vi "TrALEX_RNG.vi"(0 "Analog Amplitude":dbl=1.0 format="%0.2p", 1 "Repetition Frequency":dbl=2.0 format="%.6f") -> ()   [LabVIEW 2011]
uses:
  <vilib>/DAQmx/write.llb/DAQmx Write (Analog Wfm 1Chan NSamp).vi
  <vilib>/DAQmx/create/channels.llb/DAQmx Create Channel (AO-Voltage-Basic).vi
  <vilib>/DAQmx/configure/timing.llb/DAQmx Timing (Sample Clock).vi
  <vilib>/DAQmx/create/channels.llb/DAQmx Create Channel (CO-Pulse Generation-Frequency).vi
  <vilib>/DAQmx/configure/events/hardwareSignals.llb/DAQmx Export Signal (Most Signals).vi
  <vilib>/DAQmx/configure/trigger.llb/DAQmx Start Trigger (Digital Edge).vi
  <vilib>/DAQmx/configure/timing.llb/DAQmx Timing (Implicit).vi
  <vilib>/DAQmx/miscellaneous.llb/DAQmx Fill In Error Info.vi
  <vilib>/measure/NI_MABase.lvlib
panel:
  in  "Three Colour Duty Cycle":dbl=0.3333333333333333 format="%.6f"
  in  "Stop Button":bool
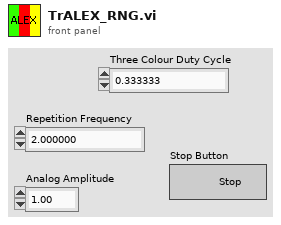
[diagram p1: front panel]
types:
  T1 = enum16{"Sine Wave", "Triangle Wave", "Square Wave", "Sawtooth Wave"}
  T2 = cluster{"Ao0 Sample Clock Rate":dbl, "Ao0 Sample Clock Rate":dbl}
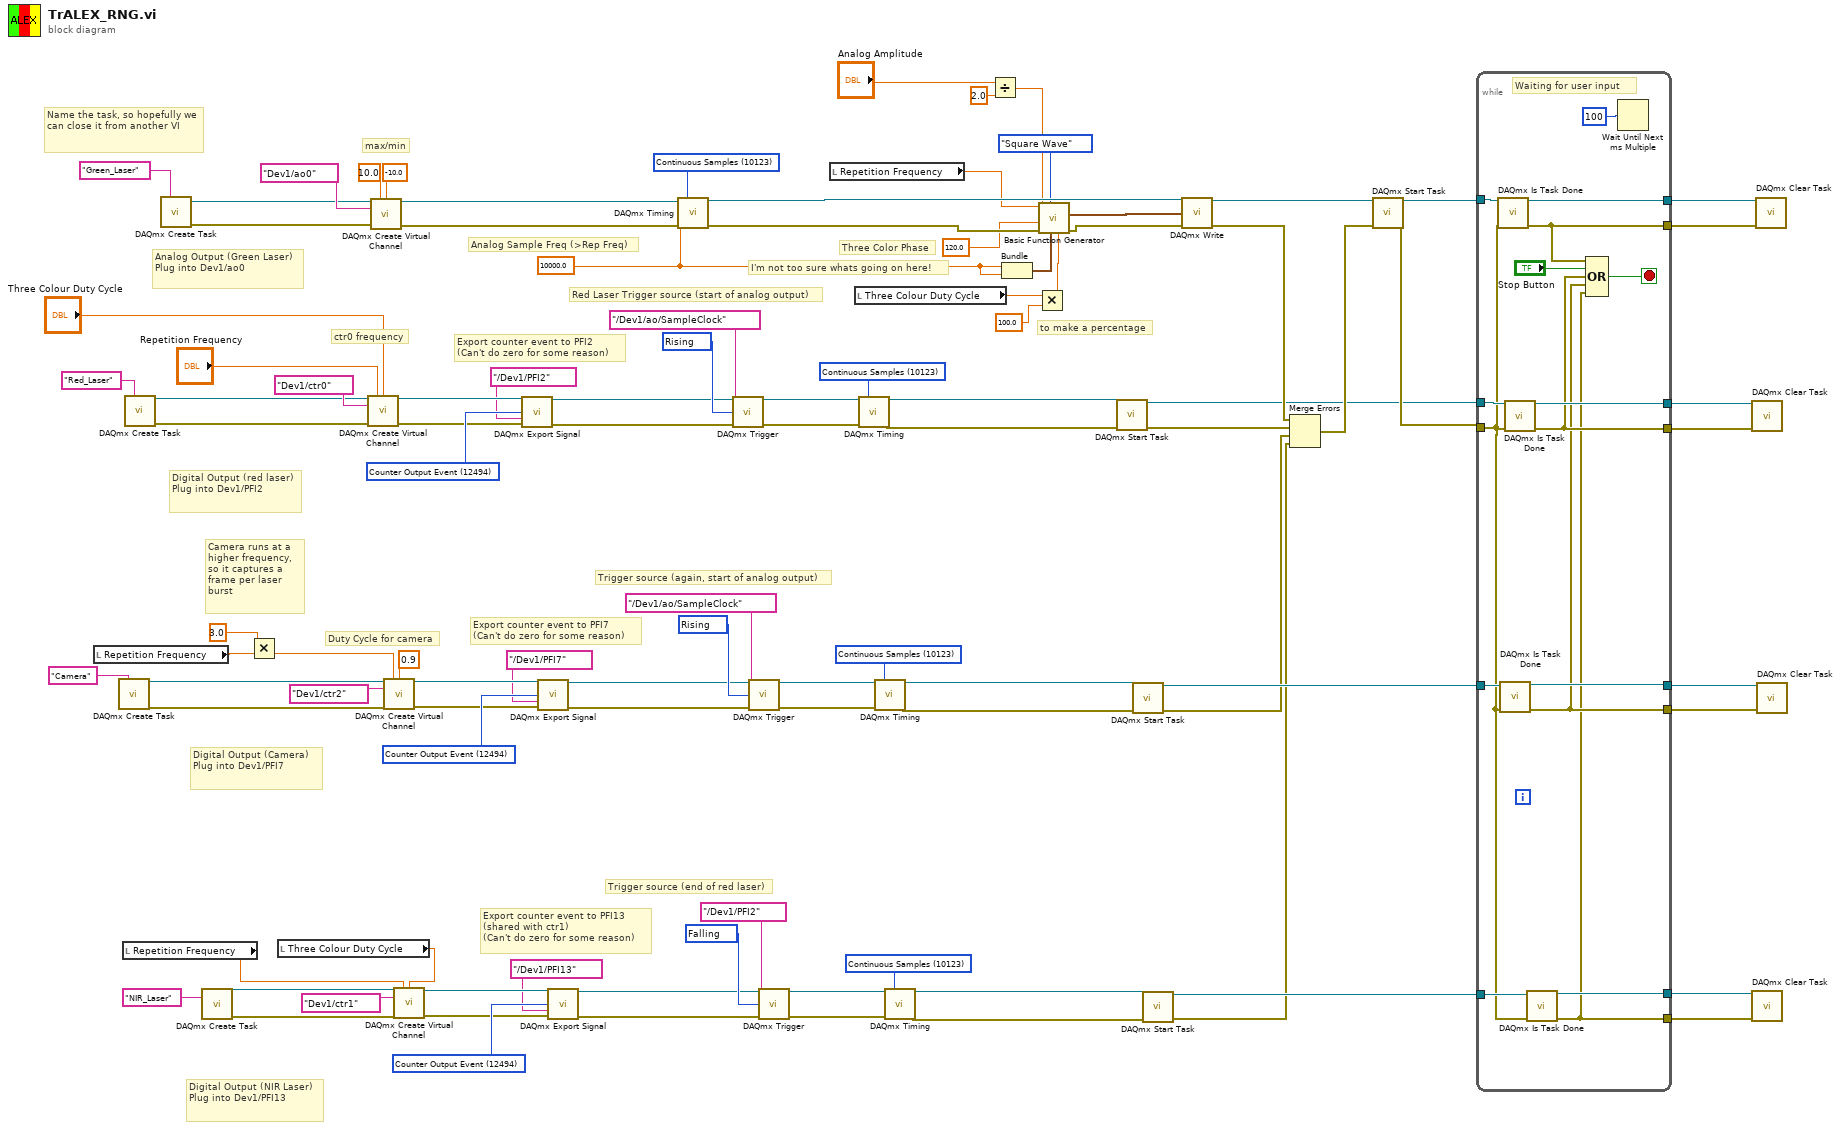
[diagram p0: block diagram]
diagram:
  w30 = 10171 items=["Rising"=10280, "Falling"=10171] ("edge")
  w33 = 10123 items=["Finite Samples"=10178, "Continuous Samples"=10123, "Hardware Timed Single Point"=12522] ("sample mode")
  w35 = 12494 items=["AI Convert Clock"=12484, "10MHz Reference Clock"=12536, "20MHz Timebase Clock"=12486, "Sample Clock"=12487, "Advance Trigger"=12488, "Reference Trigger"=12490, "Start Trigger"=12491, "Advance Complete Event"=12492, "AI Hold Complete Event"=12493, "Counter Output Event"=12494, "Change Detection Event"=12511, "Watchdog Timer Expired Event"=12512] ("signal")
  w54 = 10280 items=["Rising"=10280, "Falling"=10171] ("edge")
  w57 = 10123 items=["Finite Samples"=10178, "Continuous Samples"=10123, "Hardware Timed Single Point"=12522] ("sample mode")
  w59 = 12494 items=["AI Convert Clock"=12484, "10MHz Reference Clock"=12536, "20MHz Timebase Clock"=12486, "Sample Clock"=12487, "Advance Trigger"=12488, "Reference Trigger"=12490, "Start Trigger"=12491, "Advance Complete Event"=12492, "AI Hold Complete Event"=12493, "Counter Output Event"=12494, "Change Detection Event"=12511, "Watchdog Timer Expired Event"=12512] ("signal")
  w68 = 10123 items=["Finite Samples"=10178, "Continuous Samples"=10123, "Hardware Timed Single Point"=12522] ("sample mode")
  w89 = 10280 items=["Rising"=10280, "Falling"=10171] ("edge")
  w94 = 10123 items=["Finite Samples"=10178, "Continuous Samples"=10123, "Hardware Timed Single Point"=12522] ("sample mode")
  w96 = 12494 items=["AI Convert Clock"=12484, "10MHz Reference Clock"=12536, "20MHz Timebase Clock"=12486, "Sample Clock"=12487, "Advance Trigger"=12488, "Reference Trigger"=12490, "Start Trigger"=12491, "Advance Complete Event"=12492, "AI Hold Complete Event"=12493, "Counter Output Event"=12494, "Change Detection Event"=12511, "Watchdog Timer Expired Event"=12512] ("signal")
  w37 = 10000.0 ("Ao0 Sample Clock Rate")
  # "Name the task, so hopefully we can close it from another VI"
  # "to make a percentage"
  # "Digital Output (NIR Laser) Plug into Dev1/PFI13"
  # "Trigger source (end of red laser)"
  # "Export counter event to PFI13 (shared with ctr1)\n(Can't do zero for some reason)"
  # "Duty Cycle for camera"
  # "Camera runs at a higher frequency, so it captures a frame per laser burst"
  # "Digital Output (Camera) Plug into Dev1/PFI7"
  # "Trigger source (again, start of analog output)"
  # "Export counter event to PFI7\n(Can't do zero for some reason)"
  # "Digital Output (red laser) Plug into Dev1/PFI2"
  # "Analog Output (Green Laser) Plug into Dev1/ao0"
  # "Three Color Phase"
  # "Analog Sample Freq (>Rep Freq)"
  # "I'm not too sure whats going on here!"
  # "Red Laser Trigger source (start of analog output)"
  # "Export counter event to PFI2\n(Can't do zero for some reason)"
  # "ctr0 frequency"
  # "max/min"
  n1 = local read "Repetition Frequency"() -> (w46:dbl)
  n2 = call <vilib>:"DAQmx Create Task.vi"("new task name"="Camera") -> ("task out"=w4:refnum<k21>, "error out"=w3:errorcluster)  [unwired: 13 in]
  n3 = local read "Repetition Frequency"() -> (w14:dbl)
  n4 = call <vilib>:"DAQmx Create Task.vi"("new task name"="Red_Laser") -> ("task out"=w6:refnum<k21>, "error out"=w5:errorcluster)  [unwired: 13 in]
  n5 = call <vilib>:"DAQmx Create Task.vi"("new task name"="Green_Laser") -> ("task out"=w12:refnum<k21>, "error out"=w11:errorcluster)  [unwired: 13 in]
  n6 = call <vilib>:"DAQmx Create Task.vi"("new task name"="NIR_Laser") -> ("task out"=w2:refnum<k21>, "error out"=w1:errorcluster)  [unwired: 13 in]
  n7 = Multiply(x=3.0 ("Repetition Frequency"), y=w46) -> (x*y=w45:dbl)
  n8 = local read "Three Colour Duty Cycle"() -> (w18:dbl)
  n9 = call-poly <vilib>:"DAQmx Create Virtual Channel.vi"("task in"=w6, "frequency"="Repetition Frequency", "duty cycle"="Three Colour Duty Cycle", "counter"=tag "Dev1/ctr0", "error in"=w5) -> ("task out"=w97:refnum<k21>, "error out"=w95:errorcluster)  [unwired: 9 in]
  n10 = call-poly <vilib>:"DAQmx Create Virtual Channel.vi"("task in"=w12, "maximum value"=10.0, "minimum value"=-10.0, "physical channels"=tag "Dev1/ao0", "error in"=w11) -> ("task out"=w101:refnum<k21>, "error out"=w100:errorcluster)  [unwired: 9 in]
  n11 = call-poly <vilib>:"DAQmx Create Virtual Channel.vi"("task in"=w4, "frequency"=w45, "duty cycle"=0.9, "counter"=tag "Dev1/ctr2", "error in"=w3) -> ("task out"=w60:refnum<k21>, "error out"=w58:errorcluster)  [unwired: 9 in]
  n12 = call-poly <vilib>:"DAQmx Create Virtual Channel.vi"("task in"=w2, "frequency"=w14, "duty cycle"=w18, "counter"=tag "Dev1/ctr1", "error in"=w1) -> ("task out"=w36:refnum<k21>, "error out"=w34:errorcluster)  [unwired: 9 in]
  n13 = call-poly <vilib>:"DAQmx Export Signal.vi"("task/channels in"=w97, "signal"=w96, "output terminal"=tag "/Dev1/PFI2", "error in"=w95) -> ("task out"=w88:refnum<k21>, "error out"=w85:errorcluster)  [unwired: 10 in]
  n14 = call-poly <vilib>:"DAQmx Export Signal.vi"("task/channels in"=w60, "signal"=w59, "output terminal"=tag "/Dev1/PFI7", "error in"=w58) -> ("task out"=w53:refnum<k21>, "error out"=w50:errorcluster)  [unwired: 10 in]
  n15 = call-poly <vilib>:"DAQmx Export Signal.vi"("task/channels in"=w36, "signal"=w35, "output terminal"=tag "/Dev1/PFI13", "error in"=w34) -> ("task out"=w29:refnum<k21>, "error out"=w26:errorcluster)  [unwired: 10 in]
  n16 = call-poly <vilib>:"DAQmx Timing.vi"("task/channels in"=w101, "sample mode"=w68, "rate"=w37, "error in"=w100) -> ("task out"=w93:refnum<k21>, "error out"=w92:errorcluster)  [unwired: 10 in]
  n17 = call-poly <vilib>:"DAQmx Trigger.vi"("task/channels in"=w88, "source"=tag "/Dev1/ao/SampleClock", "edge"=w89, "error in"=w85) -> ("task out"=w87:refnum<k21>, "error out"=w86:errorcluster)  [unwired: 10 in]
  n18 = call-poly <vilib>:"DAQmx Trigger.vi"("task/channels in"=w53, "source"=tag "/Dev1/ao/SampleClock", "edge"=w54, "error in"=w50) -> ("task out"=w52:refnum<k21>, "error out"=w51:errorcluster)  [unwired: 10 in]
  n19 = call-poly <vilib>:"DAQmx Trigger.vi"("task/channels in"=w29, "source"=tag "/Dev1/PFI2", "edge"=w30, "error in"=w26) -> ("task out"=w28:refnum<k21>, "error out"=w27:errorcluster)  [unwired: 10 in]
  n20 = local read "Repetition Frequency"() -> (w65:dbl)
  n21 = local read "Three Colour Duty Cycle"() -> (w21:dbl)
  n22 = call-poly <vilib>:"DAQmx Timing.vi"("task/channels in"=w87, "sample mode"=w94, "error in"=w86) -> ("task out"=w81:refnum<k21>, "error out"=w80:errorcluster)  [unwired: 11 in]
  n23 = call-poly <vilib>:"DAQmx Timing.vi"("task/channels in"=w52, "sample mode"=w57, "error in"=w51) -> ("task out"=w49:refnum<k21>, "error out"=w48:errorcluster)  [unwired: 11 in]
  n24 = call-poly <vilib>:"DAQmx Timing.vi"("task/channels in"=w28, "sample mode"=w33, "error in"=w27) -> ("task out"=w25:refnum<k21>, "error out"=w24:errorcluster)  [unwired: 11 in]
  n25 = Divide(x="Analog Amplitude", y=2.0) -> (x/y=w62:dbl)
  n26 = Bundle("Ao0 Sample Clock Rate"=w37, "Ao0 Sample Clock Rate"=w37) -> (w38:T2)  [unwired: 1 in]
  n27 = Multiply(x=w21, y=100.0) -> (x*y=w20:dbl)
  n28 = call <vilib>:"Basic Function Generator.vi"("offset"=w62, "square wave duty cycle (%)"=w20, "sampling info"=w38, "signal type"=T1."Square Wave", "error in (no error)"=w92, "phase"=120.0, "amplitude"=w62, "frequency"=w65) -> ("error out"=w83:errorcluster, "signal out"=w84:waveform(dbl))  [unwired: 1 in, 1 out]
  n29 = call <vilib>:"DAQmx Start Task.vi"("task/channels in"=w81, "error in"=w80) -> ("task out"=w69:refnum<k21>, "error out"=w79:errorcluster)  [unwired: 12 in]
  n30 = call <vilib>:"DAQmx Start Task.vi"("task/channels in"=w49, "error in"=w48) -> ("task out"=w42:refnum<k21>, "error out"=w41:errorcluster)  [unwired: 12 in]
  n31 = call <vilib>:"DAQmx Start Task.vi"("task/channels in"=w25, "error in"=w24) -> ("task out"=w17:refnum<k21>, "error out"=w13:errorcluster)  [unwired: 12 in]
  n32 = call-poly <vilib>:"DAQmx Write.vi"("task/channels in"=w93, "data"=w84, "error in"=w83) -> ("task out"=w76:refnum<k21>, "error out"=w78:errorcluster)  [unwired: 10 in, 1 out]
  n33 = Merge Errors(w78, w79, w41, w13) -> (w77:errorcluster)
  n34 = call <vilib>:"DAQmx Start Task.vi"("task/channels in"=w76, "error in"=w77) -> ("task out"=w75:refnum<k21>, "error out"=w74:errorcluster)  [unwired: 12 in]
  n35 = while {
    tunnel: [w118] -> w70
    tunnel: [w111] -> w73
    tunnel: [w115] -> w71
    tunnel: [w109] -> w72
    tunnel: w75 -> [w114]
    tunnel: w74 -> [w103]
    tunnel: w69 -> [w113]
    tunnel: w42 -> [w112]
    tunnel: [w108] -> w40
    tunnel: [w107] -> w39
    tunnel: w17 -> [w106]
    tunnel: [w105] -> w16
    tunnel: [w104] -> w15
    stop <- w116 stop-if-true
    # "Waiting for user input"
    n36 = call <vilib>:"DAQmx Is Task Done.vi"("task/channels in"=w114, "error in"=w103) -> ("task out"=w118:refnum<k21>, "error out"=w111:errorcluster)  [unwired: 11 in, 1 out]
    n37 = call <vilib>:"DAQmx Is Task Done.vi"("task/channels in"=w112, "error in"=w103) -> ("task out"=w108:refnum<k21>, "error out"=w107:errorcluster)  [unwired: 11 in, 1 out]
    n38 = call <vilib>:"DAQmx Is Task Done.vi"("task/channels in"=w113, "error in"=w103) -> ("task out"=w115:refnum<k21>, "error out"=w109:errorcluster)  [unwired: 11 in, 1 out]
    n39 = call <vilib>:"DAQmx Is Task Done.vi"("task/channels in"=w106, "error in"=w103) -> ("task out"=w105:refnum<k21>, "error out"=w104:errorcluster)  [unwired: 11 in, 1 out]
    n40 = Compound Arithmetic op=OR(w111, "Stop Button", w109, w107, w104) -> (w116:bool)
    n41 = Wait Until Next ms Multiple(millisecond multiple=u32 100) -> ()  [unwired: 1 out]
  }
  n42 = call <vilib>:"DAQmx Clear Task.vi"("task in"=w71, "error in"=w72) -> ()  [unwired: 13 in, 1 out]
  n43 = call <vilib>:"DAQmx Clear Task.vi"("task in"=w16, "error in"=w15) -> ()  [unwired: 13 in, 1 out]
  n44 = call <vilib>:"DAQmx Clear Task.vi"("task in"=w70, "error in"=w73) -> ()  [unwired: 13 in, 1 out]
  n45 = call <vilib>:"DAQmx Clear Task.vi"("task in"=w40, "error in"=w39) -> ()  [unwired: 13 in, 1 out]
